vi "Configure Amplitude Characteristics.vi"(0 "VISA resource name":refnum<visa-resource-name>, 1 "Maximum Mixer Power (-10 dBm)":dbl=-10.0, 2 "External Amplifier Gain (0 dB)":dbl, 3 "IF Gain (0: Auto)":u16(ring) items=["Auto", "Fixed"], 5 "Enable Presel Center (T: Enable)":bool=TRUE, 7 "Presel Adjust (0 Hz)":dbl, 9 "Enable Internal Preamp (T: Enable)":bool=TRUE, 11 "error in (no error)":errorcluster, 12 "Enable Microwave Preselector (T: Enable)":bool=TRUE, 13 "Preselector (0: MWave)":u16(ring) items=["MWave", "MMWave", "External"]) -> (4 "VISA resource name out":refnum<visa-resource-name>, 15 "error out":errorcluster)   [LabVIEW 2014, in "Agilent ESA PSA Series.lvlib"]
doc: "Configures Internal Preamp and Preselector."
uses:
  Agilent ESA PSA Series.lvlib
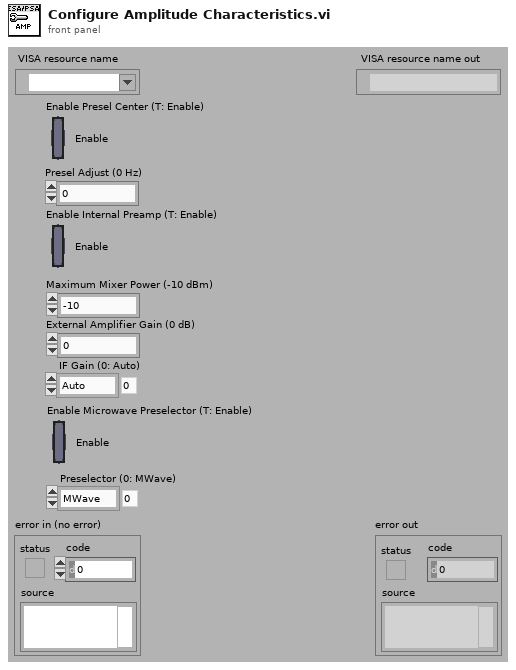
[diagram p1: front panel]
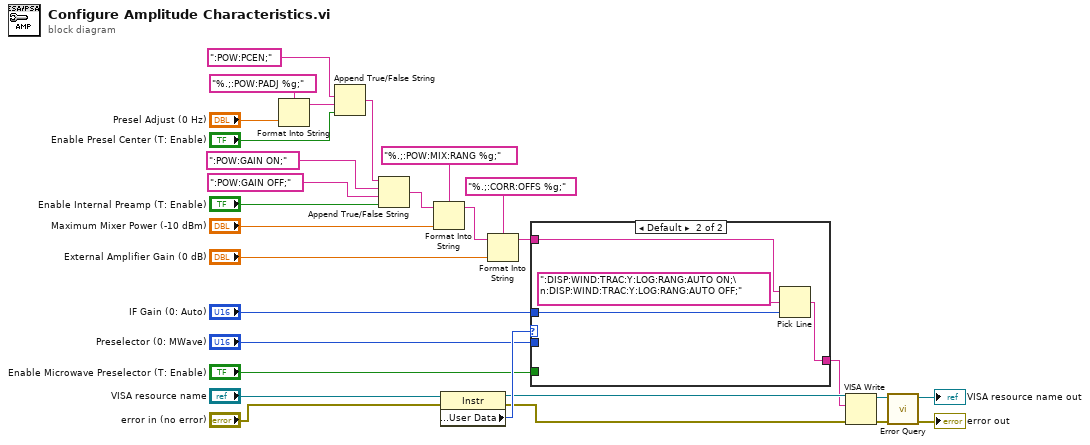
[diagram p0: block diagram]
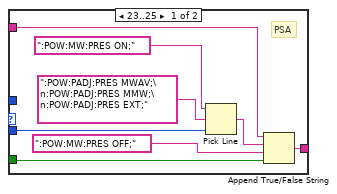
[diagram p2: hidden frame]
diagram:
  n1 = Format Into String(format string="%.;:POW:PADJ %g;" ("true string"), "Presel Adjust (0 Hz)") -> (resulting string=w21:string)  [unwired: 2 in, 1 out]
  n2 = Append True/False String(1:"Enable Presel Center (T: Enable)", 2:w21, 3:":POW:PCEN;" ("true string")) -> (0:w3:string)  [unwired: 1 in]
  n3 = Append True/False String(1:"Enable Internal Preamp (T: Enable)", 2:":POW:GAIN OFF;" ("true string"), 3:":POW:GAIN ON;" ("true string"), 4:w3) -> (0:w17:string)
  n4 = Format Into String(format string="%.;:POW:MIX:RANG %g;", initial string=w17, "Maximum Mixer Power (-10 dBm)") -> (resulting string=w12:string)  [unwired: 1 in, 1 out]
  n5 = property on="Property Node" class="Instr"(reference="VISA resource name", error in="error in (no error)") -> (reference out=w9:refnum<visa-resource-name>, error out=w7:errorcluster, "General Settings:User Data"=w11:u32)
  n6 = Format Into String(format string="%.;:CORR:OFFS %g;", initial string=w12, "External Amplifier Gain (0 dB)") -> (resulting string=w2:string)  [unwired: 1 in, 1 out]
  n7 = case shown="Default" w11 {
    tunnel: "Enable Microwave Preselector (T: Enable)" -> [w37 _]
    tunnel: "Preselector (0: MWave)" -> [w30 _]
    tunnel: "IF Gain (0: Auto)" -> [_ w39]
    tunnel: [w35 w40] -> w1
    tunnel: w2 -> [w34 w38]
    frame 23..25 {
      # "PSA"
      n8 = Pick Line(string ("")=":POW:MW:PRES ON;" ("true string"), multi-line string=":POW:PADJ:PRES MWAV;\n:POW:PADJ:PRES MMW;\n:POW:PADJ:PRES EXT;", line index=w30) -> (output string=w32:string)
      n9 = Append True/False String(1:w37, 2:":POW:MW:PRES OFF;" ("true string"), 3:w32, 4:w34) -> (0:w35:string)
    }
    frame Default {
      n10 = Pick Line(string ("")=w38, multi-line string=":DISP:WIND:TRAC:Y:LOG:RANG:AUTO ON;\n:DISP:WIND:TRAC:Y:LOG:RANG:AUTO OFF;", line index=w39) -> (output string=w40:string)
    }
  }
  n11 = VISA Write(VISA resource name=w9, write buffer=w1, error in (no error)=w7) -> (VISA resource name out=w29:refnum<visa-resource-name>, error out=w27:errorcluster)  [unwired: 1 out]
  n12 = call "Error Query.vi"("error in (no error)"=w27, "VISA resource name"=w29) -> ("error out"=→"error out":errorcluster, "VISA resource name out"=→"VISA resource name out":refnum<visa-resource-name>)  [unwired: 6 in, 2 out]
